vi "Index Texture.vi"(7 "data value reference":refnum<data-value>, 11 "Point In Texture":T1) -> (3 "Colour":u32(colorbox))   [LabVIEW 2022 SP3, in "Raster.lvlib"]
uses:
  Raster.lvlib
  Point 2D.ctl
panel:
  in  "Use Texture (T)":bool=TRUE
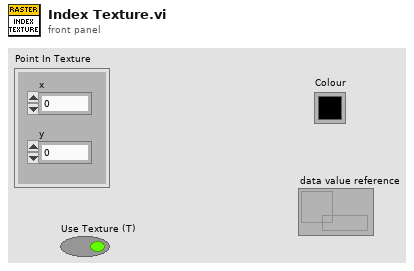
[diagram p1: front panel]
types:
  T1 = typedef "Raster.lvlib/Point 2D.ctl" = cluster{"x":i32, "y":i32}
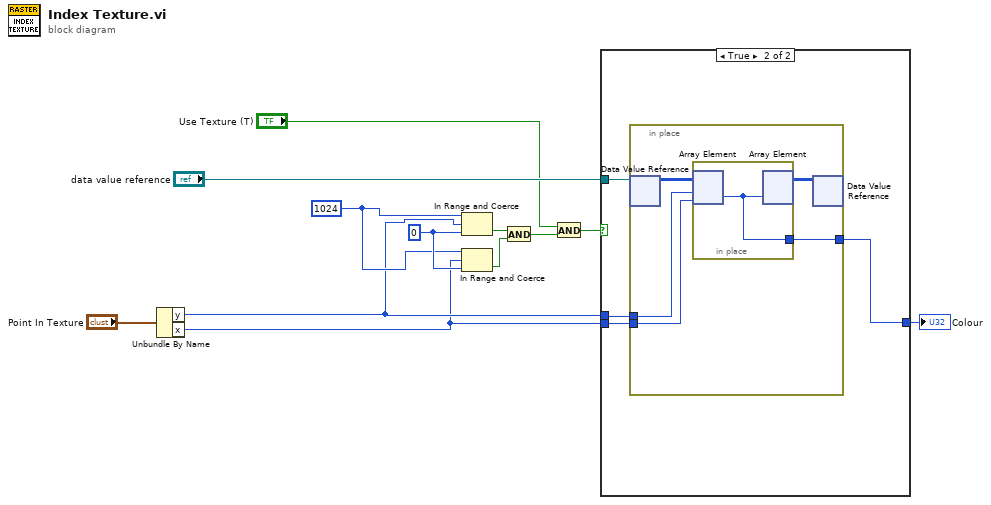
[diagram p0: block diagram]
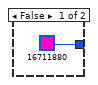
[diagram p2: hidden frame]
diagram:
  w7 = 1024 ("number of rows")
  w12 = 0 ("lower limit")
  n1 = Unbundle By Name("Point In Texture") -> ("y"=w2:i32, "x"=w1:i32)
  n2 = In Range and Coerce(upper limit=w7, x=w2, lower limit=w12) -> (In Range?=w11:bool)  [unwired: 1 out]
  n3 = In Range and Coerce(upper limit=w7, x=w1, lower limit=w12) -> (In Range?=w10:bool)  [unwired: 1 out]
  n4 = And(x=w11, y=w10) -> (x .and. y?=w5:bool)
  n5 = And(x="Use Texture (T)", y=w5) -> (x .and. y?=w6:bool)
  n6 = case shown="True" w6 {
    tunnel: w2 -> [_ w16]
    tunnel: w1 -> [_ w15]
    tunnel: [u32 16711880 w14] -> w9
    tunnel: "data value reference" -> [_ w17]
    frame False {
    }
    frame True {
      n7 = in-place {
        in-place-border: w16 -> [w21]
        in-place-border: w15 -> [w19]
        in-place-border: [w18] -> w14
        n8 = in-place-dvr #1(w17) -> (w22:u32[][])  [unwired: 1 out]
        n9 = in-place {
          in-place-border: [w23] -> w18
          n10 = in-place-array #2(w22, w21, w19) -> (w23:u32)
          n11 = in-place-array #2(w23) -> (w20:u32[][])  [unwired: 2 out]
        }
        n12 = in-place-dvr #1(w20) -> ()  [unwired: 2 out]
      }
    }
  }
  "Colour" <- w9
